vi "GEN2_Bulk_Stat.vi"(5 "YOLO?":bool, 6 "Stat_to_Read":T1[](array[typedef]) items=["Torque Enable", "Homing Complete", "Goal Id", "Goal Iq", "Goal Velo", "Goal Posi", "Present Id", "Present Iq", "Present Velo", "Present Posi", "Bus Voltage", "Temperature Winding", "Temperature MOSFET", "Temperature IC", "Error Status", "Iq_Temps"], 7 "IDs":u8[](array[numeric]), 8 "error in (no error)":errorcluster, 9 "Data_to_Write":dbl[][](array[numeric]), 10 "Stat_to_Write":T1[](array[typedef]) items=["Torque Enable", "Homing Complete", "Goal Id", "Goal Iq", "Goal Velo", "Goal Posi", "Present Id", "Present Iq", "Present Velo", "Present Posi", "Bus Voltage", "Temperature Winding", "Temperature MOSFET", "Temperature IC", "Error Status", "Iq_Temps"], 11 "VISA Refnum in":refnum<visa-resource-name>) -> (0 "error out":errorcluster, 1 "ERROR":u8[](array[numeric]), 2 "Data_2D":dbl[][](array[numeric]), 3 "VISA Refnum out":refnum<visa-resource-name>)   [LabVIEW 2016, in "GEN_2.lvlib"]
uses:
  GEN_2.lvlib
  GEN2_Instructions.ctl
  GEN2_Stat_Addr.ctl
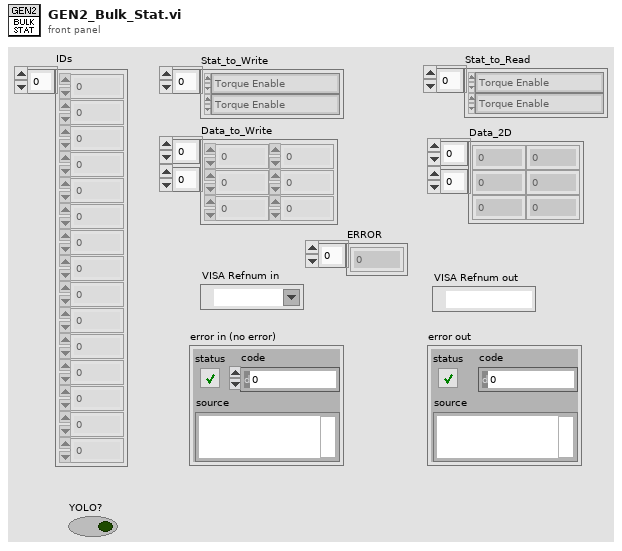
[diagram p1: front panel]
types:
  T1 = typedef "GEN_2.lvlib/GEN2_Stat_Addr.ctl" = u8
  T2 = enum16{"big-endian, network order", "native, host order", "little-endian"}
  T3 = typedef "GEN_2.lvlib/GEN2_Instructions.ctl" = u8
  T4 = cluster{"ID":u8, "ERROR":u8, "ChechSumError?":bool, "Data":string}
  T5 = cluster{"ID":u8, "ERROR":u8, "ChechSumError?":bool, "Data":string}[]
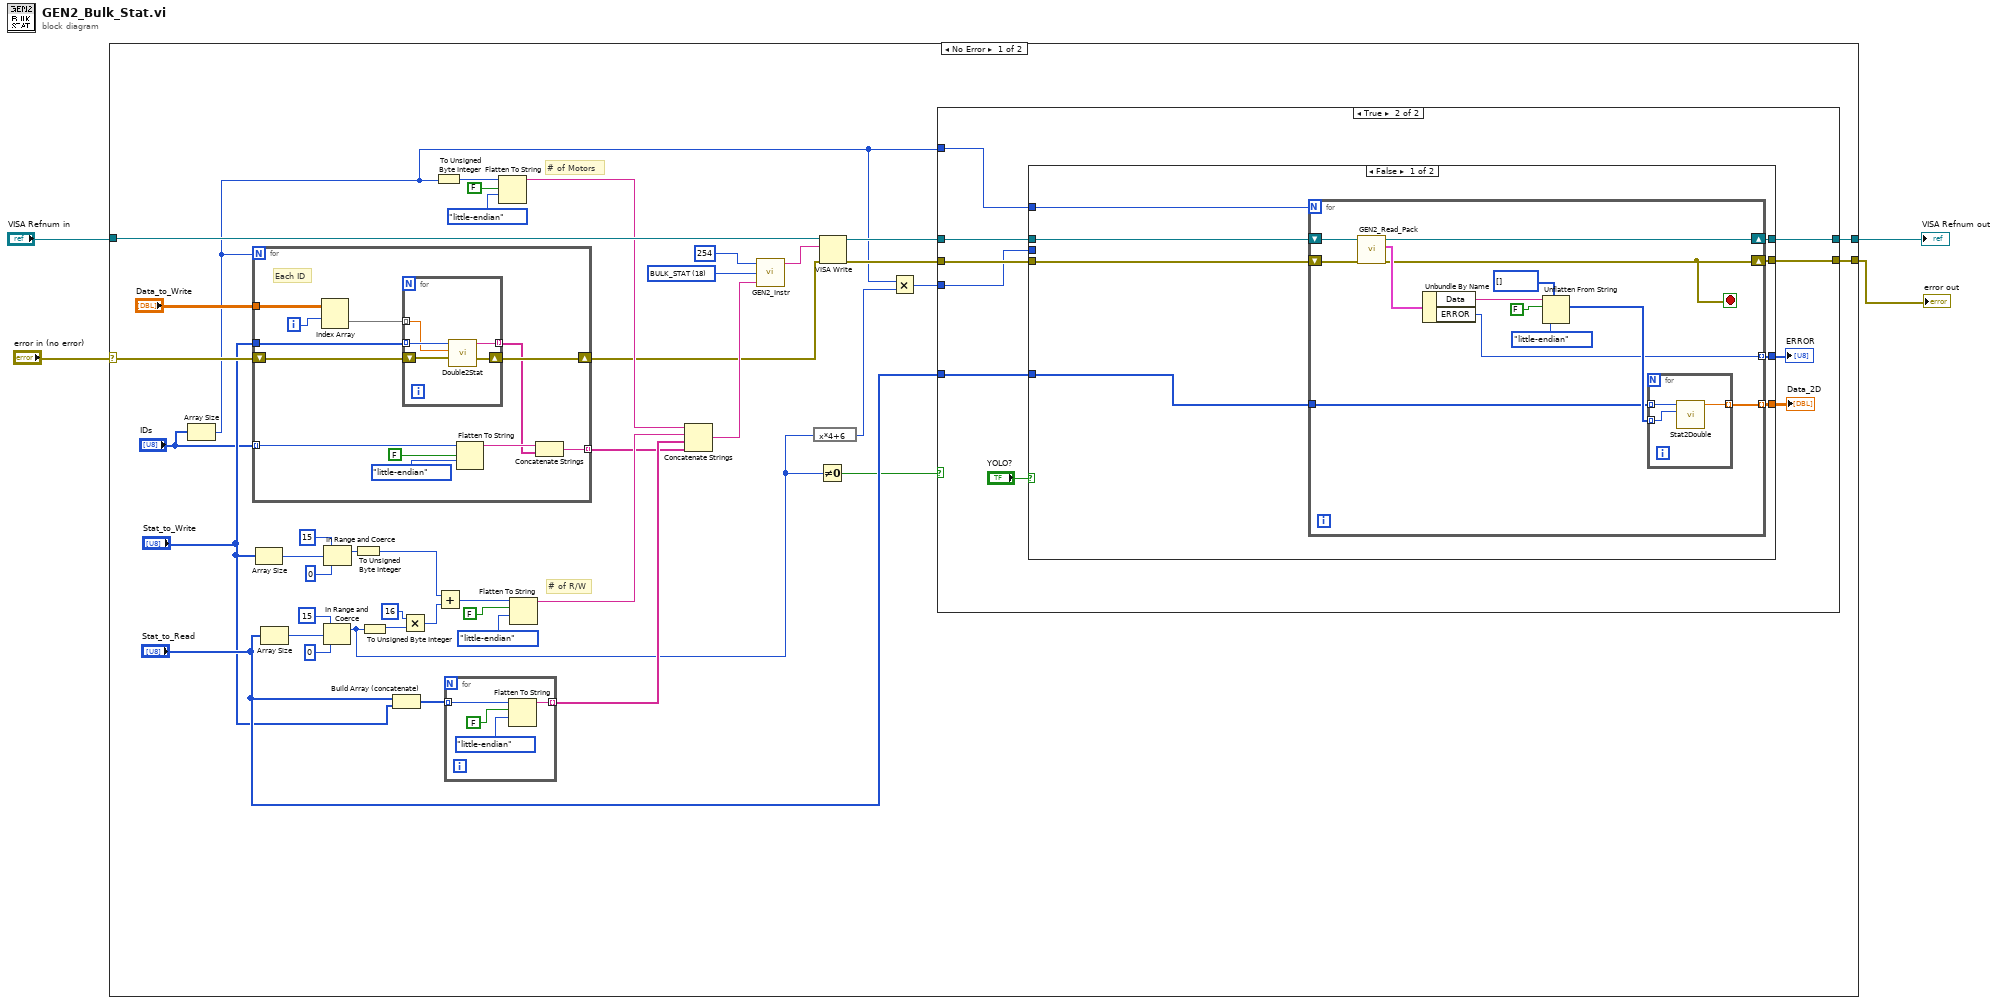
[diagram p0: block diagram]
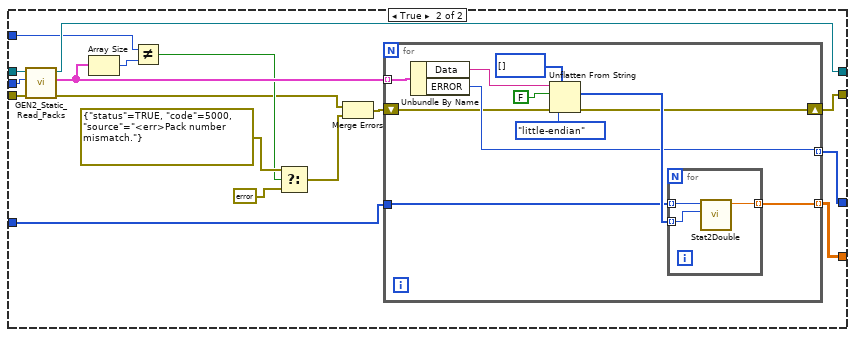
[diagram p3: hidden frame]
diagram:
  n1 = case shown="No Error" "error in (no error)" {
    selector: "error in (no error)" -> [w45 w136]
    tunnel: [w42 w135] -> w4
    tunnel: [w10 w136] -> w3
    tunnel: "VISA Refnum in" -> [w46 w135]
    frame No Error {
      w13 = T3 18 items=["PING"=1, "READ_STAT"=2, "WRITE_STAT"=3, "READ_CONFIG"=4, "WRITE_CONFIG"=5, "SAVE_CONFIG"=6, "SET_POSI"=8, "BULK_STAT"=18] ("Instruction")
      # "# of R/W"
      # "# of Motors"
      n2 = Array Size(array="IDs") -> (size(s)=w8:i32)
      n3 = for {
        N: w8 -> [_]
        tunnel: "Stat_to_Write" -> [w123]
        shift-right: [w125] -> w12
        shift-left: w45 -> [w124]
        tunnel: "Data_to_Write" -> [w116]
        tunnel: "IDs" -> [w120] mode=indexing
        tunnel: [w117] -> w16 mode=indexing
        i -> [w115]
        # "Each ID"
        n4 = Index Array(array=w116, index (row)=w115) -> (element=w114:dbl[])  [unwired: 1 in]
        n5 = for {
          tunnel: w123 -> [w130] mode=indexing
          shift-right: [w128] -> w125
          shift-left: w124 -> [w129]
          tunnel: w114 -> [w127] mode=indexing
          tunnel: [w126] -> w118 mode=indexing
          n6 = call "Double2Stat.vi"("error in (no error)"=w129, "Data"=w127, "Stat Address"=w130) -> ("error out"=w128:errorcluster, "data string"=w126:string)  [unwired: 7 in]
        }
        n7 = Flatten To String(anything=w120, prepend array or string size? (T)=FALSE, byte order (0:big-endian, network order)=T2."little-endian") -> (data string=w119:string)  [unwired: 1 in, 2 out]
        n8 = Concatenate Strings(w119, w118) -> (w117:string)
      }
      n9 = Array Size(array="Stat_to_Write") -> (size(s)=w38:i32)
      n10 = Array Size(array="Stat_to_Read") -> (size(s)=w32:i32)
      n11 = In Range and Coerce(upper limit=15, x=w32, lower limit=0) -> (coerced(x)=w6:i32)  [unwired: 1 out]
      n12 = In Range and Coerce(upper limit=15, x=w38, lower limit=0) -> (coerced(x)=w37:i32)  [unwired: 1 out]
      n13 = To Unsigned Byte Integer(number=w37) -> (unsigned 8bit integer=w23:u8)
      n14 = To Unsigned Byte Integer(number=w6) -> (unsigned 8bit integer=w31:u8)
      n15 = Build Array (concatenate)("Stat_to_Read", "Stat_to_Write") -> (w20:T1[])
      n16 = Multiply(x=u8 16, y=w31) -> (x*y=w29:u8)
      n17 = To Unsigned Byte Integer(number=w8) -> (unsigned 8bit integer=w39:u8)
      n18 = Add(x=w23, y=w29) -> (x+y=w26:u8)
      n19 = for {
        tunnel: w20 -> [w132] mode=indexing
        tunnel: [w131] -> w19 mode=indexing
        n20 = Flatten To String(anything=w132, prepend array or string size? (T)=FALSE, byte order (0:big-endian, network order)=T2."little-endian") -> (data string=w131:string)  [unwired: 1 in, 2 out]
      }
      n21 = Flatten To String(anything=w39, prepend array or string size? (T)=FALSE, byte order (0:big-endian, network order)=T2."little-endian") -> (data string=w25:string)  [unwired: 1 in, 2 out]
      n22 = Flatten To String(anything=w26, prepend array or string size? (T)=FALSE, byte order (0:big-endian, network order)=T2."little-endian") -> (data string=w24:string)  [unwired: 1 in, 2 out]
      n23 = Concatenate Strings(w25, w24, w19, w16) -> (w15:string)
      n24 = call "GEN2_Instr.vi"("Parameter"=w15, "Instruction"=w13, "ID"=u8 254) -> ("Output"=w14:string)  [unwired: 2 in]
      n25 = expression code="x*4+6"(w6) -> (w9:i32)
      n26 = Not Equal To 0?(x=w6) -> (x != 0?=w5:bool)
      n27 = VISA Write(VISA resource name=w46, write buffer=w14, error in (no error)=w12) -> (VISA resource name out=w43:refnum<visa-resource-name>, error out=w11:errorcluster)  [unwired: 1 out]
      n28 = Multiply(x=w8, y=w9) -> (x*y=w7:i32)
      n29 = case shown="True" w5 {
        tunnel: w43 -> [w48 w58]
        tunnel: [w48 w57] -> w42
        tunnel: "Stat_to_Read" -> [_ w56]
        tunnel: w11 -> [w47 w54]
        tunnel: [w47 w53] -> w10
        tunnel: w8 -> [_ w50]
        tunnel: w7 -> [_ w49]
        frame False {
        }
        frame True {
          n30 = case shown="False" "YOLO?" {
            tunnel: w58 -> [w66 w98]
            tunnel: [w65 w96] -> w57
            tunnel: w56 -> [w64 w95]
            tunnel: [w63 w94] -> w55
            tunnel: w50 -> [w62 w90]
            tunnel: w54 -> [w61 w99]
            tunnel: [w60 w97] -> w53
            tunnel: [w59 w93] -> w52
            tunnel: w49 -> [_ w83]
            frame False {
              n31 = for {
                N: w62 -> [_]
                shift-right: [w70] -> w60
                shift-left: w61 -> [w73]
                shift-right: [w71] -> w65
                shift-left: w66 -> [w72]
                tunnel: [w69] -> w63 mode=indexing
                tunnel: w64 -> [w68]
                tunnel: [w67] -> w59 mode=indexing
                stop <- w70 stop-if-true
                n32 = call "GEN2_Read_Pack.vi"("error in (no error)"=w73, "VISA Refnum in"=w72) -> ("error out"=w70:errorcluster, "Pack data"=w78:T4, "VISA Refnum out"=w71:refnum<visa-resource-name>)  [unwired: 7 in]
                n33 = Unbundle By Name(w78) -> ("Data"=w74:string, "ERROR"=w67:u8)
                n34 = Unflatten From String(type=u32[] [], binary string=w74, data includes array or string size? (T)=FALSE, byte order (0:big-endian, network order)=T2."little-endian") -> (value=w79:u32[])  [unwired: 1 in, 2 out]
                n35 = for {
                  tunnel: w68 -> [w82] mode=indexing
                  tunnel: w79 -> [w81] mode=indexing
                  tunnel: [w80] -> w69 mode=indexing
                  n36 = call "Stat2Double.vi"("Numeric in"=w81, "Stat Address"=w82) -> ("Numeric out"=w80:dbl)  [unwired: 9 in]
                }
              }
            }
            frame True {
              n37 = call "GEN2_Static_Read_Packs.vi"("error in (no error)"=w99, "byte expected"=w83, "VISA Refnum in"=w98) -> ("error out"=w85:errorcluster, "Packs"=w92:T5, "VISA Refnum out"=w96:refnum<visa-resource-name>)  [unwired: 6 in]
              n38 = Array Size(array=w92) -> (size(s)=w91:i32)
              n39 = Not Equal?(x=w90, y=w91) -> (x != y?=w86:bool)
              n40 = Select(t=errorcluster {"status"=TRUE, "code"=5000, "source"="<err>Pack number mismatch."} ("FF"), s=w86, f=errorcluster {"status"=FALSE, "code"=0, "source"=""}) -> (s? t:f=w89:errorcluster)
              n41 = Merge Errors(w85, w89) -> (w84:errorcluster)
              n42 = for {
                tunnel: w92 -> [w105] mode=indexing
                tunnel: [w104] -> w93 mode=indexing
                tunnel: [w103] -> w94 mode=indexing
                tunnel: w95 -> [w102]
                shift-right: [w100] -> w97
                shift-left: w84 -> [w101]
                n43 = Unbundle By Name(w105) -> ("Data"=w106:string, "ERROR"=w104:u8)
                n44 = Unflatten From String(type=u32[] [], binary string=w106, data includes array or string size? (T)=FALSE, byte order (0:big-endian, network order)=T2."little-endian", error in (no error)=w101) -> (value=w110:u32[], error out=w100:errorcluster)  [unwired: 1 out]
                n45 = for {
                  tunnel: w102 -> [w113] mode=indexing
                  tunnel: w110 -> [w112] mode=indexing
                  tunnel: [w111] -> w103 mode=indexing
                  n46 = call "Stat2Double.vi"("Numeric in"=w112, "Stat Address"=w113) -> ("Numeric out"=w111:dbl)  [unwired: 9 in]
                }
              }
            }
          }
          "Data_2D" <- w55
          "ERROR" <- w52
        }
      }
    }
    frame Error {
    }
  }
  "VISA Refnum out" <- w4
  "error out" <- w3
